vi "RT Error Handler - System Health and FPGA Monitoring.vi"(4 "Output Error (FPGA)":bool, 6 "Input Error (FPGA)":bool, 8 "error in (no error)":errorcluster, 11 "Message Queue":refnum<queue>) -> (3 "dup Message Queue":refnum<queue>)   [LabVIEW 2015]
uses:
  support/Message Queue/Message Cluster.ctl
  support/Message Queue/Message Queue.lvlib
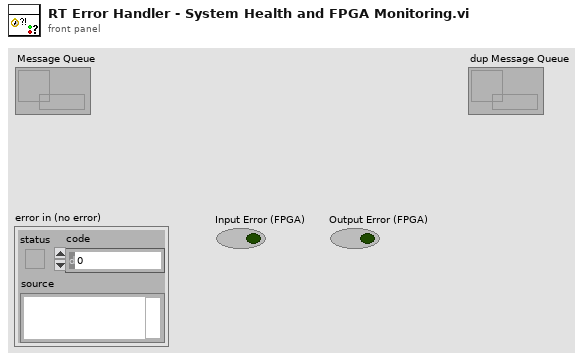
[diagram p1: front panel]
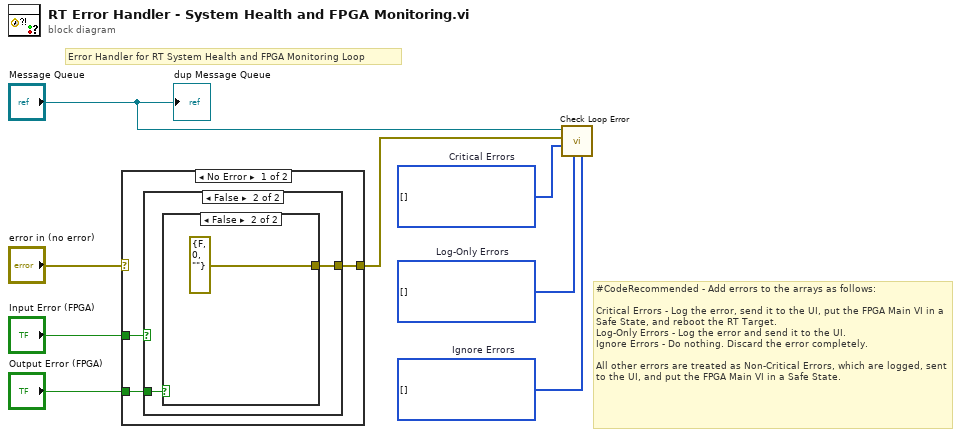
[diagram p0: block diagram]
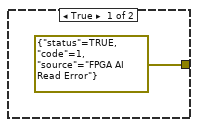
[diagram p2: hidden frame]
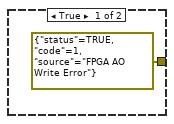
[diagram p3: hidden frame]
diagram:
  w6 = i32[] []  # Ignore Errors
  w7 = i32[] []  # Log-Only Errors
  w8 = i32[] []  # Critical Errors
  # "#CodeRecommended - Add errors to the arrays as follows:\n\nCritical Errors - Log the error, send it to the UI, put the FPGA Main VI in a Safe State, and reboot the RT Target.\nLog-Only Errors - Log the error and send it to the UI.\nIgnore Errors - Do nothing. Discard the error completely.\n\nAll other errors are treated as Non-Critical Errors, which are logged, sent to the UI, and put the FPGA Main VI in a Safe State."
  # "Error Handler for RT System Health and FPGA Monitoring Loop"
  n1 = case shown="No Error" "error in (no error)" {
    selector: "error in (no error)" -> [_ w17]
    tunnel: "Input Error (FPGA)" -> [w11 _]
    tunnel: "Output Error (FPGA)" -> [w9 _]
    tunnel: [w10 w17] -> w1
    frame No Error {
      n2 = case shown="False" w11 {
        tunnel: [errorcluster {"status"=TRUE, "code"=1, "source"="FPGA AI Read Error"} ("error constant") w14] -> w10
        tunnel: w9 -> [_ w13]
        frame True {
        }
        frame False {
          n3 = case shown="False" w13 {
            tunnel: [errorcluster {"status"=TRUE, "code"=1, "source"="FPGA AO Write Error"} ("error constant") errorcluster {"status"=FALSE, "code"=0, "source"=""} ("error constant")] -> w14
            frame True {
            }
            frame False {
            }
          }
        }
      }
    }
    frame Error {
    }
  }
  n4 = call "Check Loop Error.vi"("Ignore Errors"=w6, "Log-Only Errors"=w7, "Critical Errors"=w8, "error to process"=w1, "Message Queue"="Message Queue") -> ()  [unwired: 5 in, 2 out]
  "dup Message Queue" <- "Message Queue"
